vi "Check if Library has Changed.vi"(8 "error in (no error)":errorcluster, 10 "Test Case Path":path, 11 "Indexing Test Finder in":refnum<class "Indexing Test Finder.lvclass">) -> (0 "error out":errorcluster, 1 "Index out of date?":bool, 3 "Indexing Test Finder out":refnum<class "Indexing Test Finder.lvclass">)   [LabVIEW 2020, in "Indexing Test Finder.lvclass"]
uses:
  Indexing Test Finder.lvclass
  Indexing Test Finder.lvclass/Indexing Test Finder.ctl
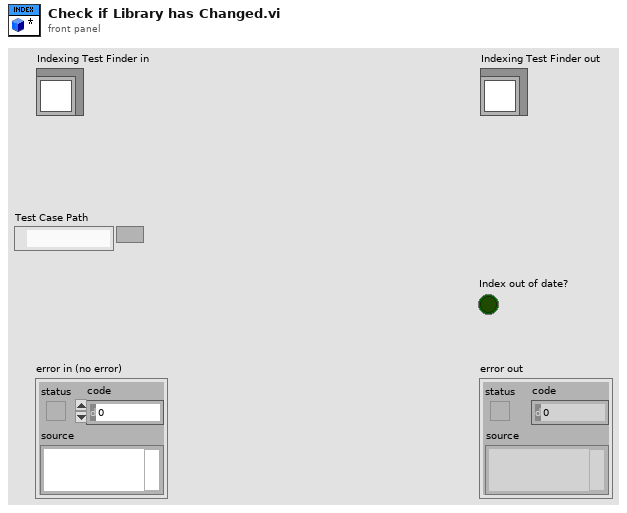
[diagram p1: front panel]
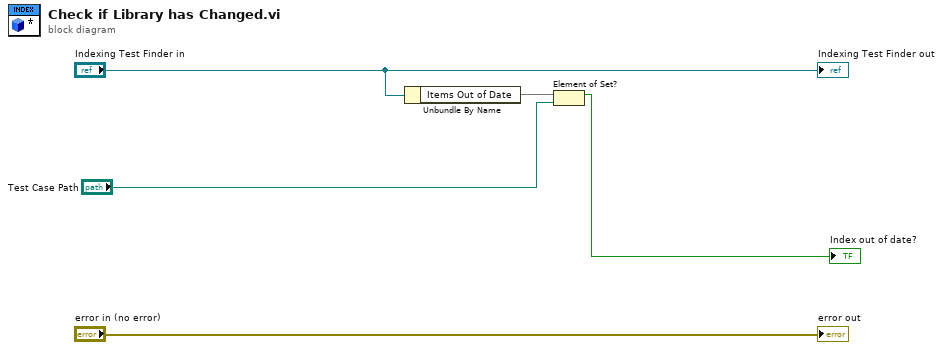
[diagram p0: block diagram]
diagram:
  n1 = Unbundle By Name("Indexing Test Finder in") -> ("Items Out of Date"=w4:set{path})
  n2 = Element of Set?(10:"Test Case Path", 11:w4) -> (3:→"Index out of date?":bool)
  "error out" <- "error in (no error)"
  "Indexing Test Finder out" <- "Indexing Test Finder in"
